vi "Save-image-of-selected-cameras.vi"(4 "Image file type":enum16{"JPG", "BMP", "PNG"}(ring), 6 "Cameras":i32, 7 "Storage directory":path, 8 "error in":errorcluster, 9 "Camera suffix":string[](array[string]), 10 "Filename":string, 11 "Image references":T1[](array[typedef])) -> (0 "error IO":errorcluster)   [LabVIEW 2013, in "CameraVision.lvlib" / "CV-Storage.lvclass"]
uses:
  CV-Storage.lvclass
  <vilib>/vision/Image Controls.llb/IMAQ Image.ctl
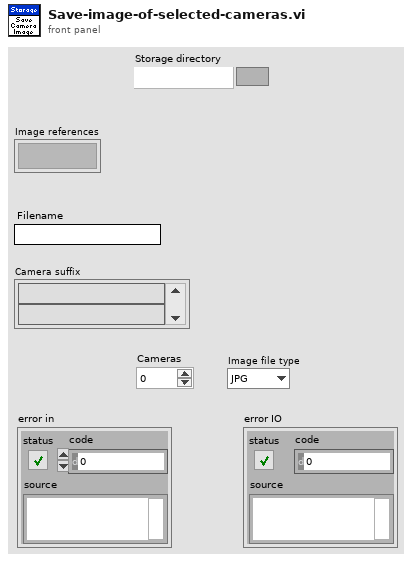
[diagram p1: front panel]
types:
  T1 = typedef "IMAQ Image.ctl" = refnum<image>
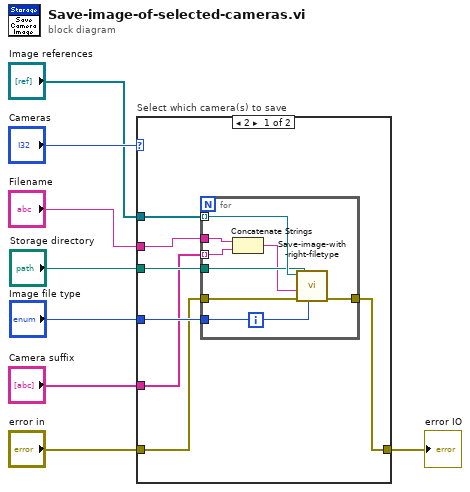
[diagram p0: block diagram]
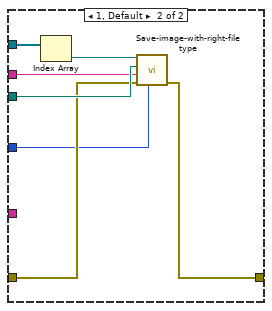
[diagram p2: hidden frame]
diagram:
  n1 = case "Select which camera(s) to save" shown="2" "Cameras" {
    tunnel: "Image file type" -> [w14 w25]
    tunnel: "Storage directory" -> [w11 w30]
    tunnel: [w12 w29] -> w1
    tunnel: "error in" -> [w13 w28]
    tunnel: "Image references" -> [w15 w27]
    tunnel: "Filename" -> [w10 w24]
    tunnel: "Camera suffix" -> [w9 _]
    frame 2 {
      n2 = for {
        tunnel: w15 -> [w21] mode=indexing
        tunnel: w14 -> [w19]
        tunnel: w13 -> [w23]
        tunnel: [w22] -> w12
        tunnel: w9 -> [w18] mode=indexing
        tunnel: w11 -> [w20]
        tunnel: w10 -> [w16]
        n3 = Concatenate Strings(w16, w18) -> (w17:string)
        n4 = call "Save-image-with-right-filetype.vi"("Image file type"=w19, "error in"=w23, "Filename"=w17, "Filepath and name"=w20, "Image in"=w21) -> ("error IO"=w22:errorcluster)  [unwired: 6 in]
      }
    }
    frame 1, Default {
      n5 = Index Array(array=w27) -> (element=w26:T1)  [unwired: 1 in]
      n6 = call "Save-image-with-right-filetype.vi"("Image file type"=w25, "error in"=w28, "Filename"=w24, "Filepath and name"=w30, "Image in"=w26) -> ("error IO"=w29:errorcluster)  [unwired: 6 in]
    }
  }
  "error IO" <- w1
